vi "Save All This Project.vi"(8 "error in (no error)":errorcluster, 10 "Exclude Dependencies? (F)":bool, 11 "Project in":refnum<vi>) -> (0 "error out":errorcluster, 3 "Project out":refnum<vi>)   [LabVIEW 2020, in "Edit LVProj.lvlib"]
doc: "Given a project reference, this VI saves all the VIs and libraries in the project and the project itself. This is equivalent to choosing the File >> Save All (This Project) menu item."
uses:
  <vilib>/Utility/EditLVProj/Edit LVProj.lvlib
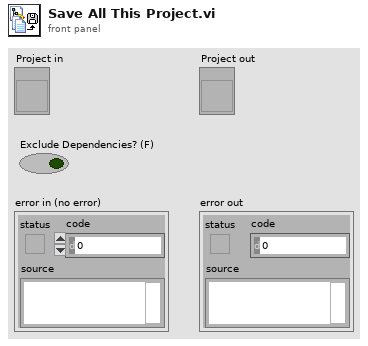
[diagram p1: front panel]
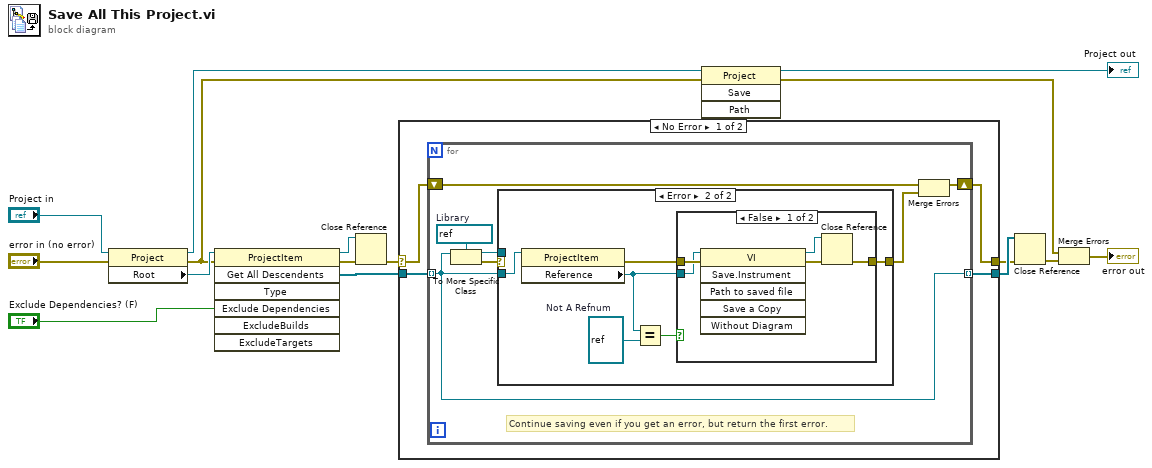
[diagram p0: block diagram]
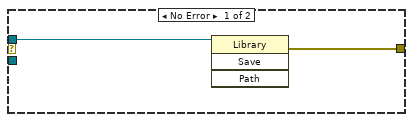
[diagram p2: hidden frame]
diagram:
  n1 = property class="Project"(reference="Project in", error in="error in (no error)") -> (reference out=w12:refnum<vi>, error out=w2:errorcluster, "Root"=w11:refnum<vi>)
  n2 = invoke class="ProjectItem" method="Get All Descendents"(reference=w11, error in=w2, "Exclude Dependencies"="Exclude Dependencies? (F)") -> (reference out=w13:refnum<vi>, error out=w14:errorcluster, "All Descendents"=w15:refnum<vi>[])  [unwired: 4 in, 4 out]
  n3 = Close Reference(reference=w13, error in (no error)=w14) -> (error out=w7:errorcluster)
  n4 = case shown="No Error" w7 {
    selector: w7 -> [w18 w42]
    tunnel: [w20 w41] -> w16
    tunnel: w15 -> [w19 w41]
    tunnel: [w17 w42] -> w6
    frame No Error {
      n5 = for {
        tunnel: w19 -> [w24] mode=indexing
        tunnel: [w24] -> w20 mode=indexing
        shift-right: [w22] -> w17
        shift-left: w18 -> [w23]
        w27 = refnum<vi> refnum  # Library
        # "Continue saving even if you get an error, but return the first error."
        n6 = To More Specific Class(target class=w27, reference=w24) -> (specific class reference=w26:refnum<vi>, error out=w25:errorcluster)  [unwired: 1 in]
        n7 = case shown="Error" w25 {
          tunnel: w26 -> [w29 _]
          tunnel: [w28 w30] -> w21
          tunnel: w24 -> [_ w34]
          frame No Error {
            n8 = invoke class="Library" method="Save"(reference=w29) -> (error out=w28:errorcluster)  [unwired: 3 in, 3 out]
          }
          frame Error {
            w33 = refnum<vi> refnum  # Not A Refnum
            n9 = property class="ProjectItem"(reference=w34) -> (error out=w35:errorcluster, "Reference"=w31:refnum<vi>)  [unwired: 1 in, 1 out]
            n10 = Equal?(x=w31, y=w33) -> (x = y?=w32:bool)
            n11 = case shown="False" w32 {
              tunnel: w35 -> [w40 _]
              tunnel: [w36 _] -> w30
              tunnel: w31 -> [w39 _]
              frame False {
                n12 = invoke class="VI" method="Save.Instrument"(reference=w39, error in=w40) -> (reference out=w38:refnum<vi>, error out=w37:errorcluster)  [unwired: 4 in, 4 out]
                n13 = Close Reference(reference=w38, error in (no error)=w37) -> (error out=w36:errorcluster)
              }
              frame True {
                # "Does not return an error\nif no VI reference available."
              }
            }
          }
        }
        n14 = Merge Errors(w23, w21) -> (w22:errorcluster)
      }
    }
    frame Error {
    }
  }
  n15 = invoke class="Project" method="Save"(reference=w12, error in=w2) -> (reference out=→"Project out":refnum<vi>, error out=w4:errorcluster)  [unwired: 2 in, 2 out]
  n16 = Close Reference(reference=w16, error in (no error)=w6) -> (error out=w5:errorcluster)
  n17 = Merge Errors(w4, w5) -> (→"error out":errorcluster)
